vi "WPI_DashboardRetrieveStatusInfo.vi"(8 "Binding Refnum":refnum<notifier>, 9 "Window Mode Notifier":refnum<notifier>, 11 "TCP Cnx":refnum<k5>) -> (0 "Power and Errors":T2, 1 "Robot Metrics":T3, 2 "Status Info":T5, 3 "Control Info":T4 {"Team Station" items=["Red 1", "Red 2", "Red 3", "Blue 1", "Blue 2", "Blue 3"]}, 4 "Robot Mode":T1(ring), 5 "Process?":bool)   [LabVIEW 2017]
uses:
  <vilib>/Rock Robotics/WPI/Dashboard/WPI_DashboardLogging Global.vi
panel:
  # "CAN Metrics\nJS HID Outputs\nFree Mem"
  # "Need to merge in TCP info too"
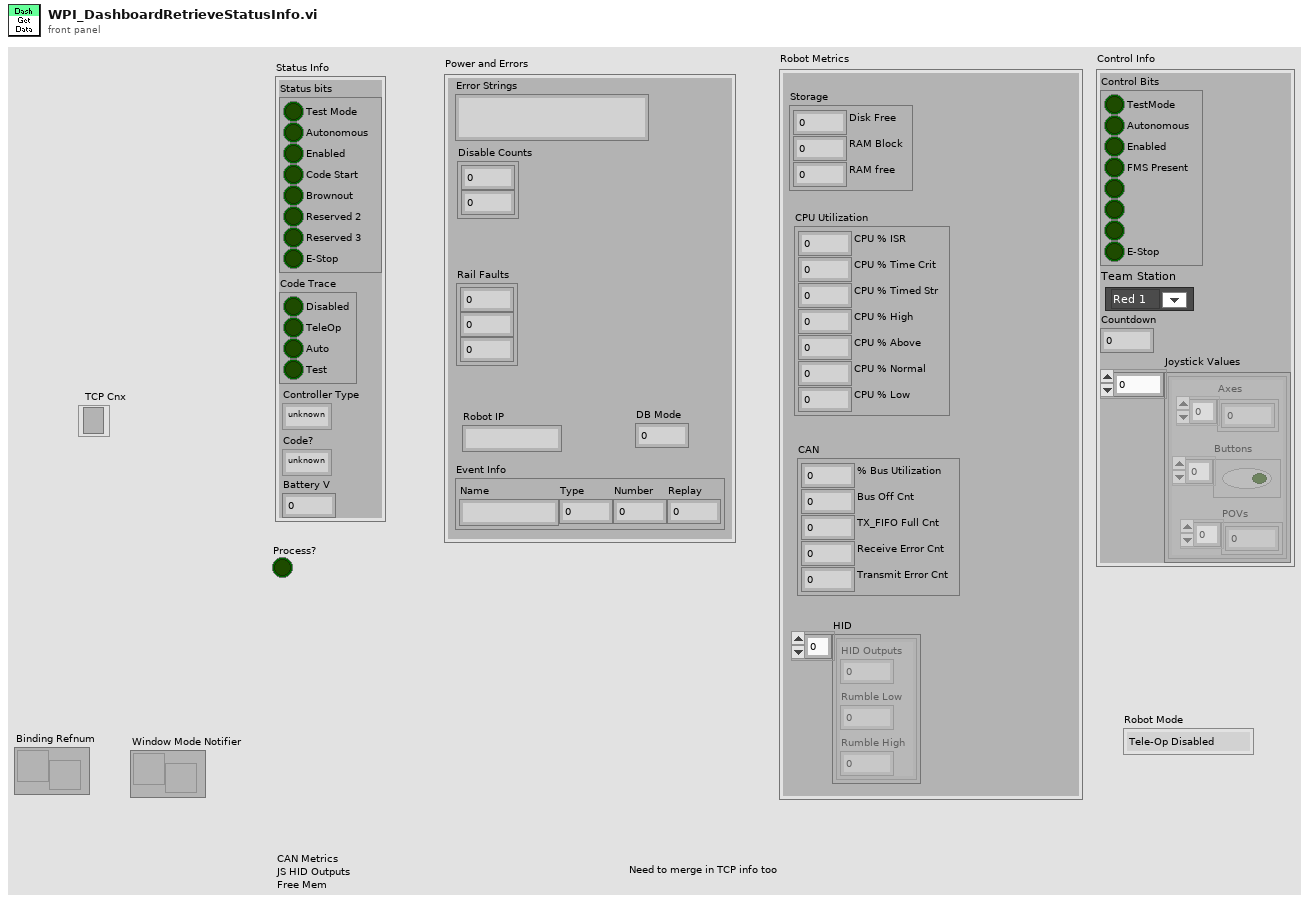
[diagram p1: front panel]
types:
  T1 = enum8{"Tele-Op Disabled", "Tele-Op Enabled", "Auto Disabled", "Auto Enabled", "Test Disabled", "Test Enabled", "Disconnected", "No Code", "E-Stop"}
  T2 = cluster{"Error Strings":string, "Disable Counts":cluster{u16, u16}, "Rail Faults":cluster{u16, u16, u16}, "Robot IP":string, "DB Mode":u8, "Event Info":cluster{"Name":string, "Type":u8, "Number":u16, "Replay":u8}}
  T3 = cluster{"Storage":cluster{"Disk Free":u64, "RAM Block":u32, "RAM free":u32}, "CPU Utilization":cluster{"CPU % ISR":sgl, "CPU % Time Crit":sgl, "CPU % Timed Str":sgl, "CPU % High":sgl, "CPU % Above":sgl, "CPU % Normal":sgl, "CPU % Low":sgl}, "CAN":cluster{"% Bus Utilization":sgl, "Bus Off Cnt":u32, "TX_FIFO Full Cnt":u32, "Receive Error Cnt":u8, "Transmit Error Cnt":u8}, "HID":cluster{"HID Outputs":u32, "Rumble Low":u16, "Rumble High":u16}[]}
  T4 = cluster{"Control Bits":cluster{"TestMode":bool, "Autonomous":bool, "Enabled":bool, "FMS Present":bool, bool, bool, bool, "E-Stop":bool}, "Team Station ":u8, "Countdown":sgl, "Joystick Values":cluster{"Axes":dbl[], "Buttons":bool[], "POVs":i16[]}[]}
  T5 = cluster{"Status bits":cluster{"Test Mode":bool, "Autonomous":bool, "Enabled":bool, "Code Start":bool, "Brownout":bool, "Reserved 2":bool, "Reserved 3":bool, "E-Stop":bool}, "Code Trace":cluster{"Disabled":bool, "TeleOp":bool, "Auto":bool, "Test":bool}, "Controller Type":enum16{"unknown", "cRIO", "roboRio"}, "Code?":enum16{"unknown", "noCode", "code"}, "Battery V":dbl}
  T6 = cluster{"TestMode":bool, "Autonomous":bool, "Enabled":bool, "FMS Present":bool, bool, bool, bool, "E-Stop":bool}
  T7 = enum16{"Standard", "Buffered", "CRLF", "Immediate"}
  T8 = cluster{"UDP Status":string, "TCP":string, "UDP Control":string}
  T9 = cluster{"Boolean array":cluster{"Boolean array[0]":bool, "Boolean array[1]":bool, "Boolean array[2]":bool, "Boolean array[3]":bool, "Boolean array[4]":bool, "Boolean array[5]":bool, "Boolean array[6]":bool, "Boolean array[7]":bool}, u8, "Countdown":sgl, cluster{dbl[], bool[], i16[]}[]}
  T10 = cluster{cluster{"Disk Free":u64, "RAM Block":u32, "RAM free":u32}, cluster{"CPU Load ISR":sgl, "CPU Load Time Critical Pr":sgl, "CPU Load Timed Str Pr":sgl, "CPU Load High Pr":sgl, "CPU Load Above Normal Pr":sgl, "CPU Load Normal Pr":sgl, "CPU Load Low Pr":sgl}, cluster{"% Bus Utilization":sgl, "Bus Off Cnt":u32, "TX_FIFO Full Cnt":u32, "Receive Error Cnt":u8, "Transmit Error Cnt":u8}, cluster{"HID Outputs":u32, "Rumble Low":u16, "Rumble High":u16}[]}
  T11 = cluster{"Status":cluster{"Test Mode":bool, "Autonomous":bool, "Enabled":bool, "Code Start":bool, "Brownout":bool, "Reserved 2":bool, "Reserved 3":bool, "E-Stop":bool}, cluster{bool, bool, bool, bool}, "ctrl":enum16{"unknown", "cRIO", "roboRio"}, "code?":enum16{"unknown", "noCode", "code"}, dbl}
  T12 = cluster{"Boolean array[0]":bool, "Boolean array[1]":bool, "Boolean array[2]":bool, "Boolean array[3]":bool, "Boolean array[4]":bool, "Boolean array[5]":bool, "Boolean array[6]":bool, "Boolean array[7]":bool}
  T13 = cluster{"Error Strings":string, "Disable Counts":cluster{u16, u16}, "Rail Faults":cluster{u16, u16, u16}, "Robot IP":string, "Mode":u8, "Event Info":cluster{"Name":string, "Type":u8, "Number":u16, "Replay":u8}}
  T14 = typedef "Protocol Operations.ctl" = enum16{"Unknown", "Keep Alive", "Client Hello", "Version not supported", "Server Hello Complete", "Assign", "Update", "No Op", "Server Hello", "Client Hello Complete", "Update Flags", "Delete Entry", "Delete All", "RPC Exec", "RPC Response"}
  T15 = typedef "Field Data.ctl" = cluster{"Dbl":dbl, "String":string, "Type":T16, "Boolean":bool, "Sequence #":T17, "Flags":u8}
  T16 = typedef "Field Type.ctl" = enum8{"Invalid", "Bool", "Numeric", "String", "Raw", "Boolean Array", "Numeric Array", "String Array", "RPC"}
  T17 = typedef "Sequence.ctl" = u16
  T18 = cluster{"Operation":T14, "Name":string, "Field Value":T15}[]
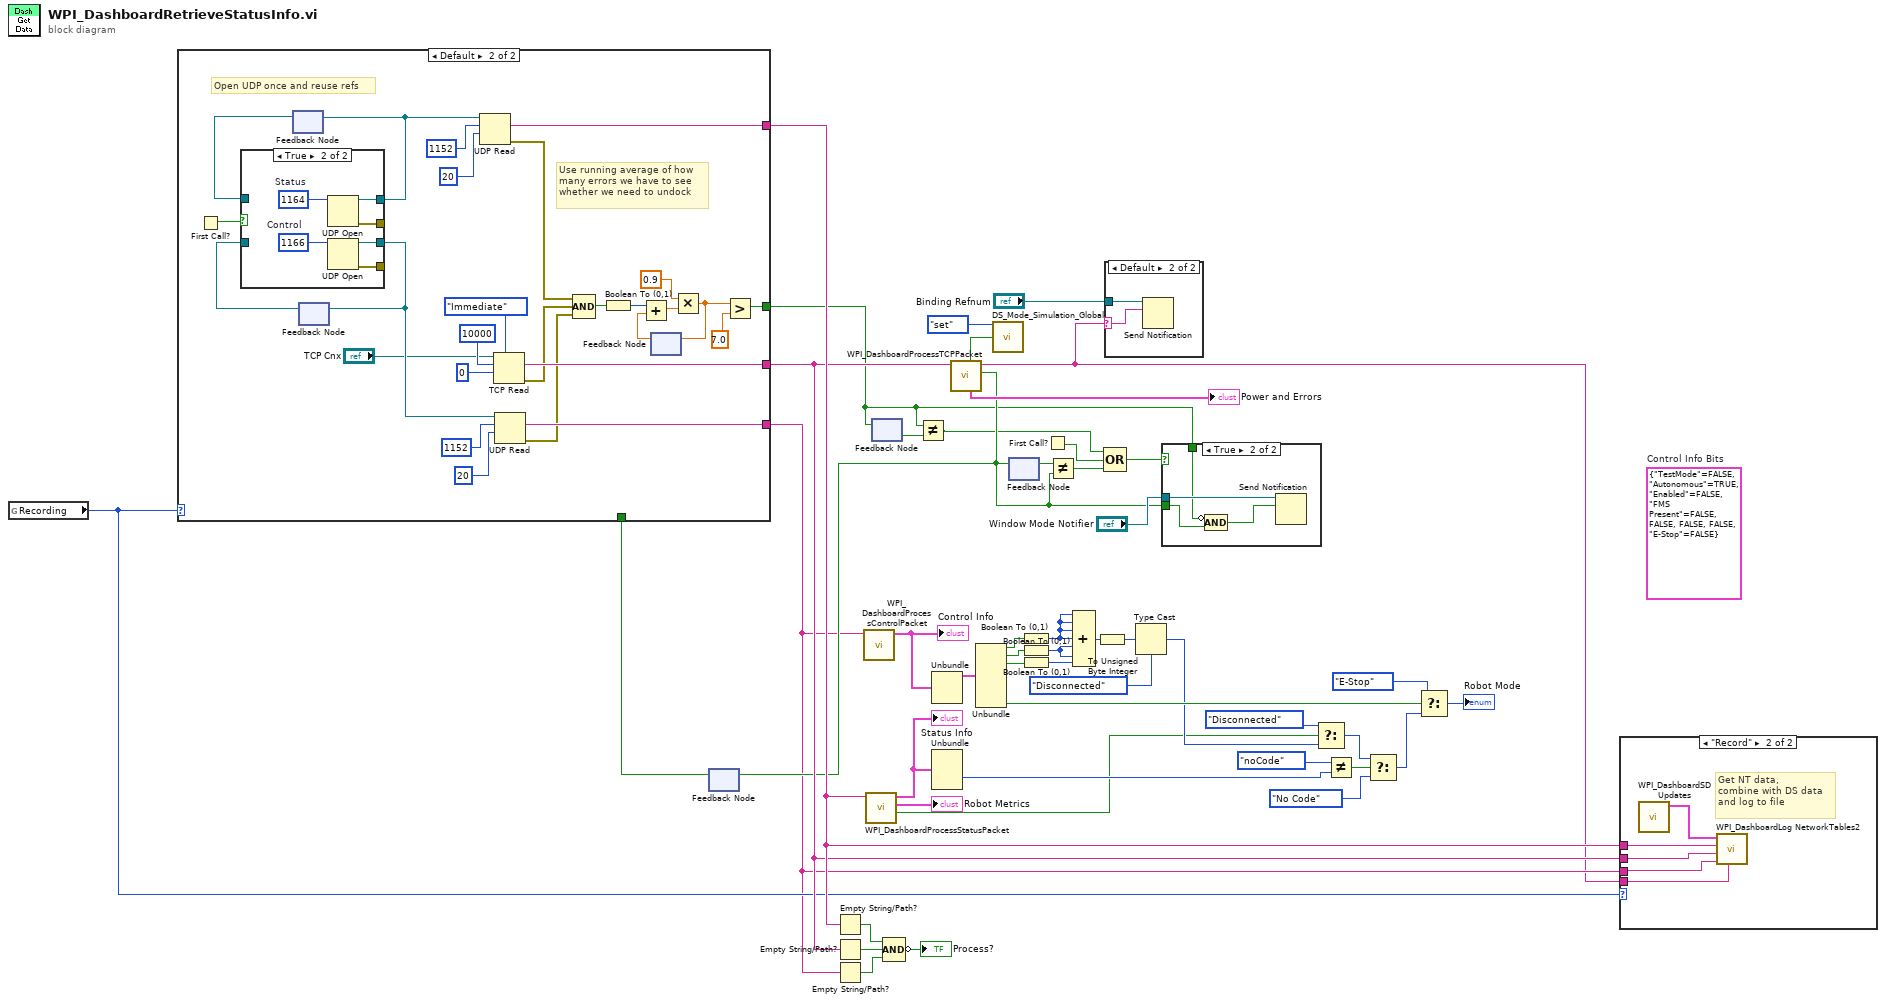
[diagram p0: block diagram]
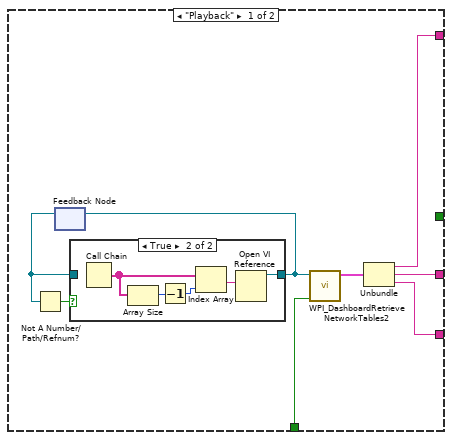
[diagram p4: hidden frame]
diagram:
  (unwired) T6 {"TestMode"=FALSE, "Autonomous"=TRUE, "Enabled"=FALSE, "FMS Present"=FALSE, FALSE, FALSE, FALSE, "E-Stop"=FALSE}  # Control Info Bits
  n1 = global read "WPI_DashboardLogging Global.vi" "Recording"() -> (w11:enum32{"Stop", "Record", "Playback"})
  n2 = feedback #1() -> (w12:bool)  [unwired: 1 in]
  n3 = case shown="Default" w11 {
    tunnel: [w51 w82] -> w7
    tunnel: [w52 w81] -> w16
    tunnel: [w50 w80] -> w15
    tunnel: w12 -> [w49 _]
    tunnel: [_ w63] -> w10
    frame "Playback" {
      n4 = feedback #2() -> (w56:refnum<vi>)  [unwired: 1 in]
      n5 = Not A Number/Path/Refnum?(number/path/refnum=w56) -> (NaN/Path/Refnum?=w55:bool)
      n6 = case shown="True" w55 {
        tunnel: w56 -> [w57 _]
        tunnel: [w57 w61] -> w53
        frame False {
        }
        frame True {
          n7 = Call Chain() -> (call chain=w60:string[])
          n8 = Array Size(array=w60) -> (size(s)=w59:i32)
          n9 = Decrement(x=w59) -> (x-1=w58:i32)
          n10 = Index Array(array=w60, index=w58) -> (element=w62:string)
          n11 = Open VI Reference(vi path=w62) -> (vi reference=w61:refnum<vi>)  [unwired: 5 in, 1 out]
        }
      }
      n12 = feedback-in #2(w53) -> ()
      n13 = call <vilib>:"WPI_DashboardRetrieve NetworkTables2.vi"("Docked Window"=w49, "DB Main Ref"=w53) -> ("Strings"=w54:T8)  [unwired: 9 in]
      n14 = Unbundle(w54) -> ("UDP Status"=w52:string, "TCP"=w50:string, "UDP Control"=w51:string)
    }
    frame Default {
      # "Use running average of how\nmany errors we have to see\nwhether we need to undock"
      # "Open UDP once and reuse refs"
      n15 = First Call?() -> (First Call?: T/F=w79:bool)
      n16 = feedback #3() -> (w77:refnum<k16>)  [unwired: 1 in]
      n17 = feedback #4() -> (w75:refnum<k16>)  [unwired: 1 in]
      n18 = case shown="True" w79 {
        tunnel: [w91 w95] -> w78
        tunnel: [_ w94] -> _
        tunnel: [w90 w93] -> w76
        tunnel: [_ w92] -> _
        tunnel: w77 -> [w91 _]
        tunnel: w75 -> [w90 _]
        frame False {
        }
        frame True {
          w96 = u16 1166  # Control
          w97 = u16 1164  # Status
          n19 = UDP Open(11:w97) -> (port=w95:refnum<k16>, 0:w94:errorcluster)  [unwired: 2 in, 3 out]
          n20 = UDP Open(11:w96) -> (port=w93:refnum<k16>, 0:w92:errorcluster)  [unwired: 2 in, 3 out]
        }
      }
      n21 = feedback-in #3(w78) -> ()
      n22 = feedback-in #4(w76) -> ()
      n23 = UDP Read(connection ID=w78, max size (548)=1152, timeout ms (25000)=20 ("length (rest)")) -> (data out=w81:string, error out=w73:errorcluster)  [unwired: 1 in, 3 out]
      n24 = TCP Read(connection ID="TCP Cnx", bytes to read=10000 ("timeout ms (25000)"), 7:T7."Immediate" ("mode (standard)"), 9:0 ("timeout ms (25000)")) -> (data out=w80:string, error out=w72:errorcluster)  [unwired: 1 in, 1 out]
      n25 = UDP Read(connection ID=w76, max size (548)=1152, timeout ms (25000)=20 ("length (rest)")) -> (data out=w82:string, error out=w71:errorcluster)  [unwired: 1 in, 3 out]
      n26 = Compound Arithmetic op=AND(w73, w72, w71) -> (w70:bool)
      n27 = Boolean To (0,1)(Boolean=w70) -> (0, 1=w69:i16)
      n28 = feedback #5() -> (w68:dbl)  [unwired: 1 in]
      n29 = Add(x=w69, y=w68) -> (x+y=w67:dbl)
      n30 = Multiply(x=0.9 ("timeout ms (25000)"), y=w67) -> (x*y=w65:dbl)
      n31 = feedback-in #5(w65) -> ()
      n32 = Greater?(x=w65, y=7.0 ("timeout ms (25000)")) -> (0:w63:bool)
    }
  }
  n33 = Empty String/Path?(string/path=w16) -> (empty?=w6:bool)
  n34 = Empty String/Path?(string/path=w15) -> (empty?=w5:bool)
  n35 = Empty String/Path?(string/path=w7) -> (empty?=w4:bool)
  n36 = call <vilib>:"WPI_DashboardProcessControlPacket.vi"("data in"=w7) -> ("Control Info"=w39:T9)  [unwired: 10 in]
  "Control Info" <- w39
  n37 = call <vilib>:"WPI_DashboardProcessStatusPacket.vi"("data in"=w16) -> ("Disconnected"=w19:bool, "Robot Metrics"=→"Robot Metrics":T10, "Status Cluster"=w31:T11)  [unwired: 8 in]
  "Status Info" <- w31
  n38 = feedback #6() -> (w9:bool)  [unwired: 1 in]
  n39 = feedback-in #6(w10) -> ()
  n40 = Compound Arithmetic op=AND(w6, w5, w4) -> (invert →"Process?":bool)
  n41 = Not Equal?(x=w10, y=w9) -> (x != y?=w8:bool)
  n42 = Unbundle(w39) -> ("Boolean array"=w38:T12)  [unwired: 3 out]
  n43 = Unbundle(w31) -> ("code?"=w27:enum16{"unknown", "noCode", "code"})  [unwired: 4 out]
  n44 = call <vilib>:"WPI_DashboardProcessTCPPacket.vi"("data in"=w15) -> ("Docked"=w13:bool, "Robot IP"=w1:string, "Power and Errors"=→"Power and Errors":T13, "Simulated"=w17:bool)  [unwired: 6 in, 1 out]
  n45 = feedback-in #1(w13) -> ()
  n46 = Unbundle(w38) -> ("Boolean array[0]"=w33:bool, "Boolean array[1]"=w34:bool, "Boolean array[2]"=w36:bool, "Boolean array[7]"=w30:bool)  [unwired: 4 out]
  n47 = call <vilib>:"DS_Mode_Simulation_Global.vi"("menu"=enum16{"set", "get"}."set", "simulated? in"=w17) -> ()  [unwired: 12 in, 2 out]
  n48 = feedback #7() -> (w42:bool)  [unwired: 1 in]
  n49 = feedback-in #7(w13) -> ()
  n50 = Boolean To (0,1)(Boolean=w33) -> (0, 1=w32:i16)
  n51 = Boolean To (0,1)(Boolean=w34) -> (0, 1=w35:i16)
  n52 = Boolean To (0,1)(Boolean=w36) -> (0, 1=w37:i16)
  n53 = First Call?() -> (First Call?: T/F=w44:bool)
  n54 = Not Equal?(x=w42, y=w13) -> (x != y?=w43:bool)
  n55 = Compound Arithmetic op=ADD(w32, w32, w32, w32, w35, w35, w37) -> (w23:i16)
  n56 = To Unsigned Byte Integer(number=w23) -> (unsigned 8bit integer=w18:u8)
  n57 = Compound Arithmetic op=OR(w8, w44, w43) -> (w45:bool)
  n58 = case shown="Default" w1 {
    selector: w1 -> [_ w98]
    tunnel: "Binding Refnum" -> [_ w99]
    frame "" {
    }
    frame Default {
      n59 = Send Notification(notification=w98, notifier=w99) -> ()  [unwired: 1 in, 2 out]
    }
  }
  n60 = Type Cast(type=T1."Disconnected" ("Mode"), x=w18) -> (*(type *) &x=w22:T1)
  n61 = case shown="True" w45 {
    tunnel: "Window Mode Notifier" -> [_ w103]
    tunnel: w13 -> [_ w101]
    tunnel: w10 -> [_ w102]
    frame False {
    }
    frame True {
      n62 = Compound Arithmetic op=AND(invert w102, w101) -> (w100:bool)
      n63 = Send Notification(notification=w100, notifier=w103) -> ()  [unwired: 1 in, 2 out]
    }
  }
  n64 = Select(t=T1."Disconnected" ("Mode"), s=w19, f=w22) -> (s? t:f=w3:T1)
  n65 = Not Equal?(x=enum16{"unknown", "noCode", "code"}."noCode" ("code?"), y=w27) -> (x != y?=w26:bool)
  n66 = Select(t=w3, s=w26, f=T1."No Code" ("Mode")) -> (s? t:f=w25:T1)
  n67 = Select(t=T1."E-Stop" ("Mode"), s=w30, f=w25) -> (s? t:f=→"Robot Mode":T1)
  n68 = case shown="\"Record\"" w11 {
    tunnel: w16 -> [_ w105]
    tunnel: w15 -> [_ w106]
    tunnel: w7 -> [_ w107]
    tunnel: w1 -> [_ w104]
    frame Default {
    }
    frame "Record" {
      # "Get NT data,\ncombine with DS data\nand log to file"
      n69 = call <vilib>:"WPI_DashboardSD Updates.vi"() -> ("Collected Data"=w108:T18)  [unwired: 11 in]
      n70 = call <vilib>:"WPI_DashboardLog NetworkTables2.vi"("Robot IP"=w104, "UDP Control"=w107, "TCP"=w106, "UDP Status"=w105, "NT Data Values"=w108) -> ()  [unwired: 7 in]
    }
  }
